vi "Configure Trigger Mode.vi"(7 "Analog Noise Reject (T: True)":bool, 8 "error in (no error)":errorcluster, 9 "Trigger Modifier (0: No Trigger Modifier)":u16(ring) items=["No Trigger Modifier", "Auto"], 10 "Trigger Holdoff (50e-9)":dbl, 11 "VISA resource name":refnum<visa-resource-name>) -> (0 "error out":errorcluster, 3 "VISA resource name out":refnum<visa-resource-name>)   [LabVIEW 2009, in "Agilent 8000 Series.lvlib"]
doc: "Configures the trigger mode of an oscilloscope. You can configure holdoff type, Trigger Modifier and Analog Noise Reject."
uses:
  Agilent 8000 Series.lvlib
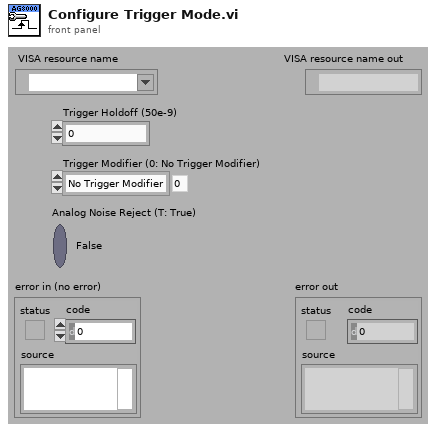
[diagram p1: front panel]
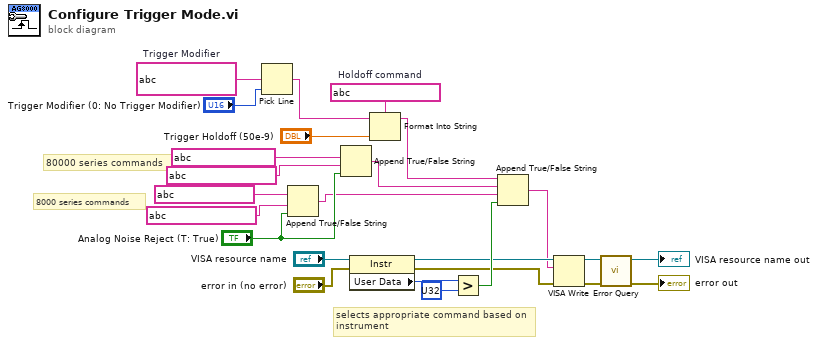
[diagram p0: block diagram]
diagram:
  w18 = string ?  # Holdoff command
  w21 = string ?  # Trigger Modifier
  # "selects appropriate command based on instrument"
  # "8000 series commands"
  # "80000 series commands"
  n1 = Pick Line(multi-line string=w21, line index="Trigger Modifier (0: No Trigger Modifier)") -> (output string=w15:string)  [unwired: 1 in]
  n2 = Append True/False String(1:"Analog Noise Reject (T: True)", 2:string ? ("Trigger Modifier"), 3:string ? ("Trigger Modifier")) -> (0:w6:string)  [unwired: 1 in]
  n3 = Append True/False String(1:"Analog Noise Reject (T: True)", 2:string ? ("Trigger Modifier"), 3:string ? ("Trigger Modifier")) -> (0:w7:string)  [unwired: 1 in]
  n4 = property class="Instr"(reference="VISA resource name", error in="error in (no error)") -> (reference out=w4:refnum<visa-resource-name>, error out=w3:errorcluster, "User Data"=w10:u32)
  n5 = Format Into String(format string=w18, initial string=w15, "Trigger Holdoff (50e-9)") -> (resulting string=w8:string)  [unwired: 1 in, 1 out]
  n6 = Greater?(x=w10, y=u32 ?) -> (0:w5:bool)
  n7 = Append True/False String(1:w5, 2:w6, 3:w7, 4:w8) -> (0:w2:string)
  n8 = VISA Write(VISA resource name=w4, write buffer=w2, error in (no error)=w3) -> (VISA resource name out=w23:refnum<visa-resource-name>, error out=w22:errorcluster)  [unwired: 1 out]
  n9 = call "Error Query.vi"("error in (no error)"=w22, "VISA resource name"=w23) -> ("error out"=→"error out":errorcluster, "VISA resource name out"=→"VISA resource name out":refnum<visa-resource-name>)  [unwired: 6 in, 2 out]
